vi "Parse Smart Syntax Representation.vi"(0 "functionbase in":refnum<class "functionbase.lvclass">, 11 "error in (no error)":errorcluster) -> (4 "functionbase out":refnum<class "functionbase.lvclass">, 6 "Scan Syntax List":T1[](array[typedef]), 8 "Smart Syntax Representation List":string[](array[string]), 15 "error out":errorcluster)   [LabVIEW 2019, in "LSL.lvlib" / "functionbase.lvclass"]
uses:
  functionbase.lvclass
  common/function utils/Scan Syntax Format.ctl
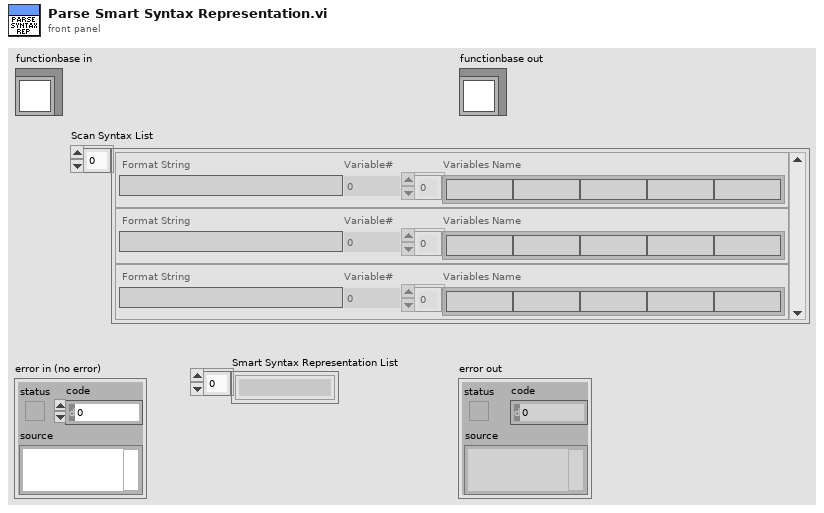
[diagram p1: front panel]
types:
  T1 = typedef "Scan Syntax Format.ctl" = cluster{"Format String":string, "Variable#":i32, "Variables Name":string[]}
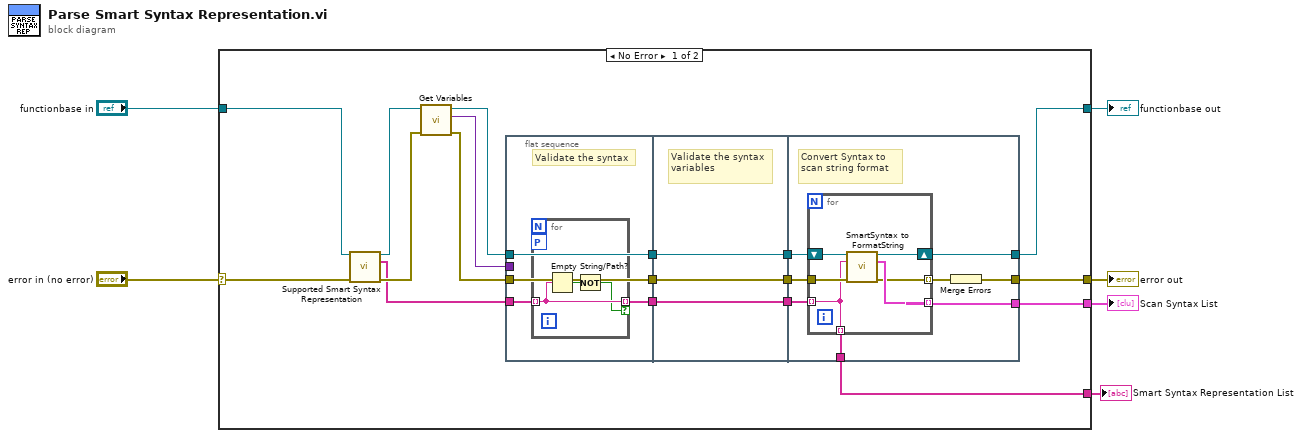
[diagram p0: block diagram]
diagram:
  n1 = case shown="No Error" "error in (no error)" {
    selector: "error in (no error)" -> [w23 w50]
    tunnel: [w9 w50] -> w5
    tunnel: [w8 w49] -> w3
    tunnel: "functionbase in" -> [w24 w49]
    tunnel: [w17 _] -> w2
    tunnel: [w7 _] -> w1
    frame No Error {
      n2 = call-dynamic "Supported Smart Syntax Representation.vi"("functionbase in"=w24, "error in (no error)"=w23) -> ("functionbase out"=w21:refnum<class "functionbase.lvclass">, "Smart Syntax Representation List"=w18:string[], "error out"=w22:errorcluster)  [unwired: 11 in]
      n3 = call-dynamic "Get Variables.vi"("error in (no error)"=w22, "functionbase in"=w21) -> ("error out"=w11:errorcluster, "Variables"=w10:variant, "functionbase out"=w16:refnum<class "functionbase.lvclass">)  [unwired: 7 in]
      n4 = flat-sequence {
        tunnel: w18 -> [w26]
        tunnel: [w25] -> w20
        tunnel: w16 -> [w28]
        tunnel: [w28] -> w15
        tunnel: [w27] -> w12
        tunnel: w11 -> [w27]
        tunnel: w10 -> [_]
        tunnel: w20 -> [w34]
        tunnel: [w34] -> w19
        tunnel: w15 -> [w33]
        tunnel: [w33] -> w14
        tunnel: [w32] -> w13
        tunnel: w12 -> [w32]
        tunnel: w19 -> [w42]
        tunnel: [w41] -> w17
        tunnel: w14 -> [w40]
        tunnel: w13 -> [w39]
        tunnel: [w37] -> w9
        tunnel: [w36] -> w8
        tunnel: [w35] -> w7
        frame #0 {
          # "Validate the syntax"
          n5 = for {
            tunnel: w26 -> [w31] mode=indexing
            tunnel: [w31] -> w25 mode=indexing if=w29
            workers-P: _ -> [_]
            n6 = Empty String/Path?(string/path=w31) -> (empty?=w30:bool)
            n7 = Not(x=w30) -> (.not. x?=w29:bool)
          }
        }
        frame #1 {
          # "Validate the syntax variables"
        }
        frame #2 {
          # "Convert Syntax to scan string format"
          n8 = for {
            tunnel: w42 -> [w43] mode=indexing
            tunnel: [w45] -> w41 mode=indexing
            shift-right: [w47] -> w36
            shift-left: w40 -> [w48]
            tunnel: w39 -> [w46]
            tunnel: [w44] -> w38 mode=indexing
            tunnel: [w43] -> w35 mode=indexing
            n9 = call-dynamic "SmartSyntax to FormatString.vi"("functionbase in"=w48, "String"=w43, "error in (no error)"=w46) -> ("functionbase out"=w47:refnum<class "functionbase.lvclass">, "Scan Syntax Format"=w45:T1, "error out"=w44:errorcluster)  [unwired: 10 in]
          }
          n10 = Merge Errors(w38) -> (w37:errorcluster)
        }
      }
    }
    frame Error {
    }
  }
  "error out" <- w5
  "functionbase out" <- w3
  "Scan Syntax List" <- w2
  "Smart Syntax Representation List" <- w1
